vi "p_programTSLAspic2.vi"(9 "clockdata 2":u32[](array[numeric])=[65535, 65535, 65535, 65535, 65535, 65535, 65535, 65535, 65535, 65535, 65535, 65535, 65535, 65535, 65535, 65535, 0, 2147483648, 0, 2147483648, 0, 2147483648, 0, 2147483648, 0, 2147483648, 0, 2147483648, 0, 2147483648, 0, 2147483648, 0] format="%08x", 10 "repetitions":u32=1048575 format="%08x", 11 "pathTSFile":path=path "C:/damic/DAMIC_TIMESLICE/DamicDebugADC18test2.txt" caption="Path to timeslice file") -> (1 "outputClockData":u32[](array[numeric]), 2 "error out 2":errorcluster)   [LabVIEW 2014]
panel:
  out "clockdata 3":u32[](array[numeric])=[65535, 65535, 65535, 65535, 65535, 65535, 65535, 65535, 65535, 65535, 65535, 65535, 65535, 65535, 65535, 65535, 0, 2147483648, 0, 2147483648, 0, 2147483648, 0, 2147483648, 0, 2147483648, 0, 2147483648, 0, 2147483648, 0, 2147483648, 0] format="%08x"
  in  "clockmessagetype":u32=286331153 format="%x"
  in  "clockitems":u8=33
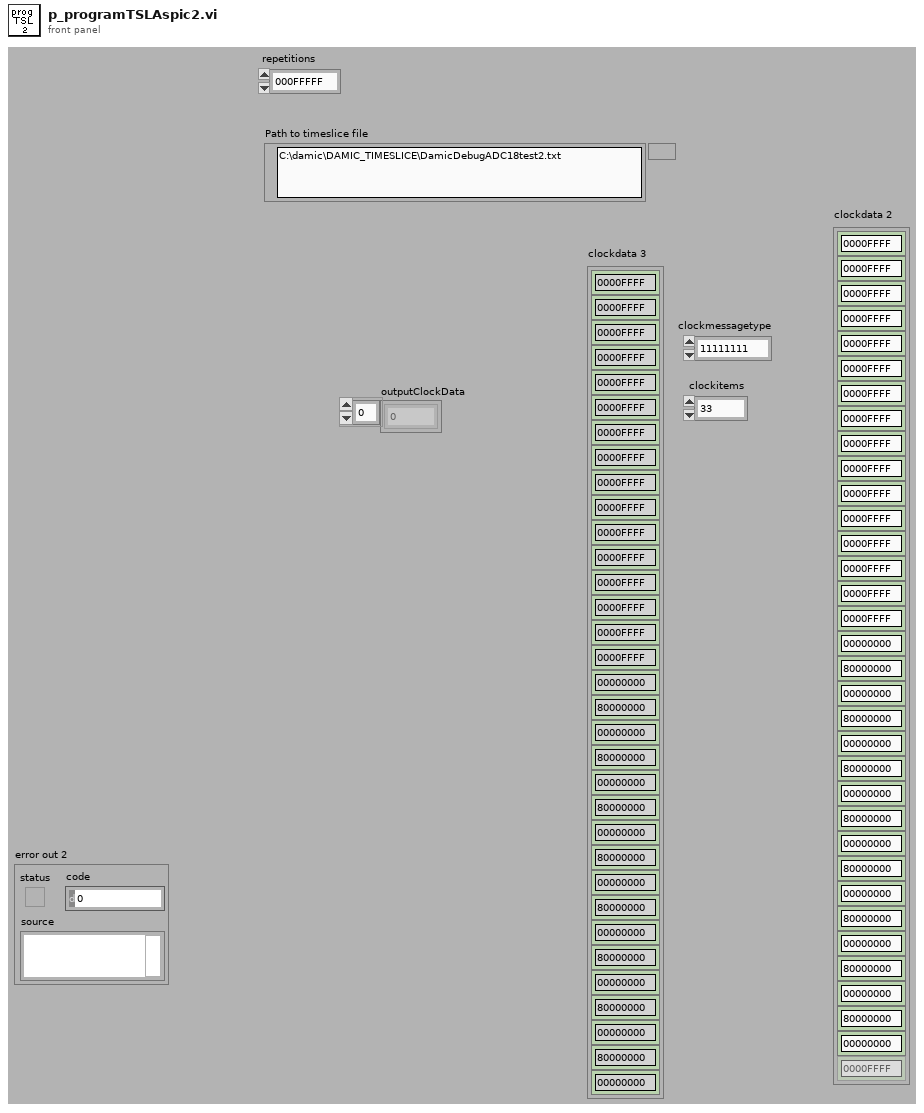
[diagram p1: front panel]
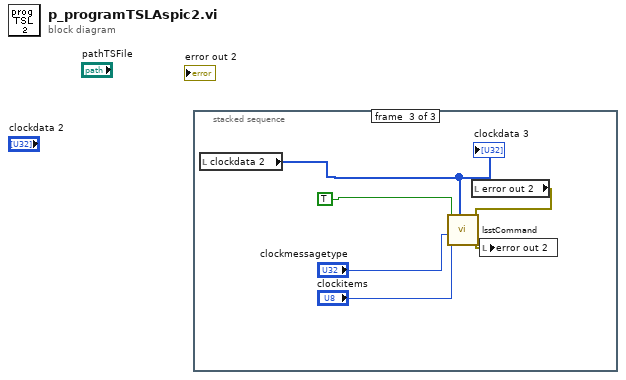
[diagram p0: block diagram]
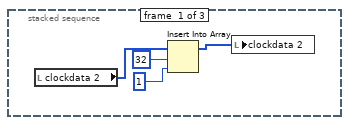
[diagram p2: hidden frame]
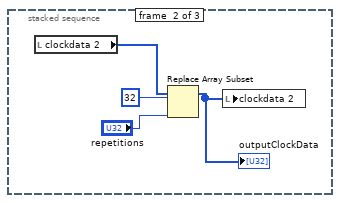
[diagram p3: hidden frame]
diagram:
  n1 = stacked-sequence {
    frame #0 {
      n2 = local read "clockdata 2"() -> (w2:u32[])
      n3 = Insert Into Array(array=w2, index=u32 32 ("numberSignals"), new element=i64 1 ("new element/subarray")) -> (w1:u32[])
      n4 = local write "clockdata 2"(w1) -> ()
    }
    frame #1 {
      n5 = local read "clockdata 2"() -> (w8:u32[])
      n6 = Replace Array Subset(array=w8, new element="repetitions", index=32) -> (w5:u32[])
      "outputClockData" <- w5
      n7 = local write "clockdata 2"(w5) -> ()
    }
    frame #2 {
      n8 = local read "clockdata 2"() -> (w9:u32[])
      "clockdata 3" <- w9
      n9 = local read "error out 2"() -> (w11:errorcluster)
      n10 = call "lsstCommand.vi"("error in (no error)"=w11, "data"=w9, "nbitems"="clockitems", "messagetype"="clockmessagetype", "execute"=TRUE) -> ("error out"=w10:errorcluster)  [unwired: 2 in, 4 out]
      n11 = local write "error out 2"(w10) -> ()
    }
  }
